vi "oa_TV Average methods(1Chan).vi"(5 "Window size":i16=10, 7 "Enum":T1(ring)=enum."Moving average", 9 "Revulotion index":i32, 10 "Angle intervals":dbl[](array[numeric]), 11 "Array":dbl[][](array[numeric])) -> (3 "Angle intervals":dbl[](array[numeric]))   [LabVIEW 2017, in "SoundVib_Torsional.lvlib"]
uses:
  <vilib>/addons/Sound and Vibration/Order Analysis/Torsional Vibration/SoundVib_Torsional.lvlib
  <vilib>/Analysis/baseanly.llb/Mean (DBL).vi
  <vilib>/Analysis/NI_AALBase.lvlib
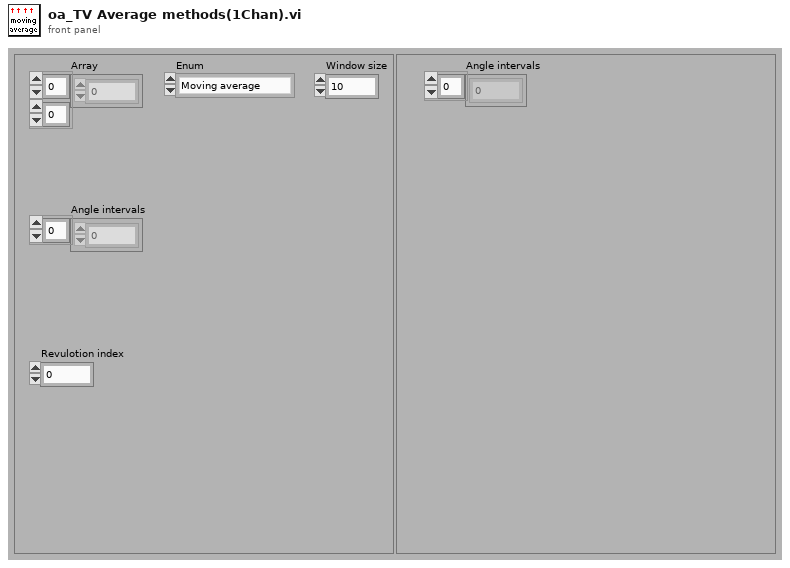
[diagram p1: front panel]
types:
  T1 = enum16{"Exponential average", "Moving average", "Current"}
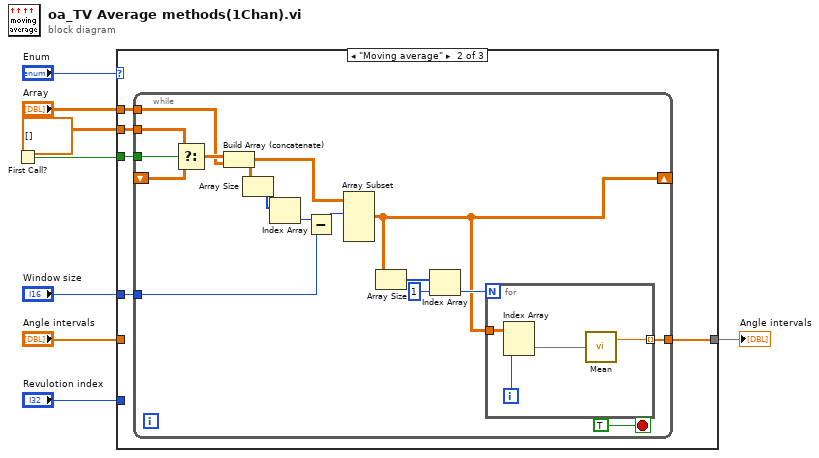
[diagram p0: block diagram]
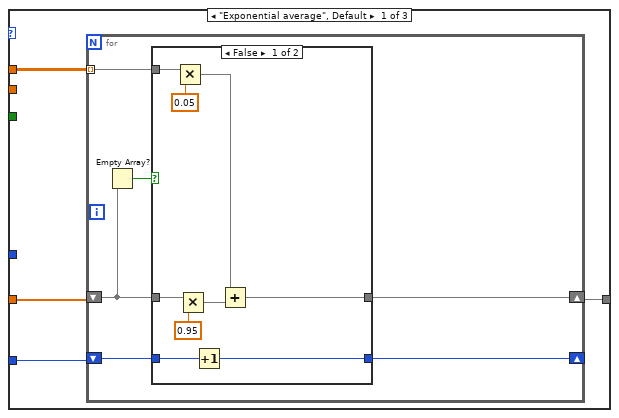
[diagram p2: hidden frame]
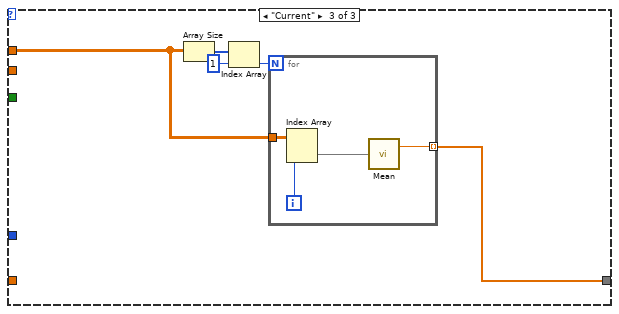
[diagram p4: hidden frame]
diagram:
  n1 = First Call?() -> (First Call?: T/F=w2:bool)
  n2 = case shown="\"Moving average\"" "Enum" {
    tunnel: "Array" -> [w12 w34 w56]
    tunnel: "Angle intervals" -> [w11 _ _]
    tunnel: [w10 w30 w55] -> w6
    tunnel: "Revulotion index" -> [w9 _ _]
    tunnel: "Window size" -> [_ w33 _]
    tunnel: w2 -> [_ w32 _]
    tunnel: dbl[][] [] ("Array") -> [_ w31 _]
    frame "Exponential average", Default {
      n3 = for {
        tunnel: w12 -> [w14] mode=indexing
        shift-right: [w17] -> _
        shift-left: w9 -> [w18]
        shift-right: [w13] -> w10
        shift-left: w11 -> [w16]
        n4 = Empty Array?(array=w16) -> (empty?=w15:bool)
        n5 = case shown="False" w15 {
          tunnel: [w19 w29] -> w13
          tunnel: w16 -> [w27 _]
          tunnel: w18 -> [w26 w28]
          tunnel: [w25 w28] -> w17
          tunnel: w14 -> [w22 w29]
          frame False {
            n6 = Multiply(x=w22, y=0.05 ("x+1")) -> (x*y=w20:dbl[])
            n7 = Multiply(x=w27, y=0.95 ("x+1")) -> (x*y=w24:dbl[])
            n8 = Increment(x=w26) -> (x+1=w25:i32)
            n9 = Add(x=w20, y=w24) -> (x+y=w19:dbl[])
          }
          frame True {
          }
        }
      }
    }
    frame "Moving average" {
      n10 = while {
        tunnel: w34 -> [w46]
        tunnel: w33 -> [w41]
        tunnel: w32 -> [w50]
        tunnel: w31 -> [w49]
        shift-right: [w36] -> _
        shift-left: _ -> [w48]
        tunnel: [w35] -> w30
        stop <- TRUE stop-if-true
        n11 = Select(t=w49, s=w50, f=w48) -> (s? t:f=w47:dbl[][])
        n12 = Build Array (concatenate)(w47, w46) -> (w44:dbl[][])
        n13 = Array Size(array=w44) -> (size(s)=w43:i32[])
        n14 = Index Array(array=w43) -> (element=w42:i32)  [unwired: 1 in]
        n15 = Subtract(x=w42, y=w41) -> (x-y=w40:i32)
        n16 = Array Subset(array=w44, index (row)=w40) -> (w36:dbl[][])  [unwired: 3 in]
        n17 = Array Size(array=w36) -> (size(s)=w39:i32[])
        n18 = Index Array(array=w39, index=1) -> (element=w37:i32)
        n19 = for {
          N: w37 -> [_]
          tunnel: w36 -> [w54]
          tunnel: [w51] -> w35 mode=indexing
          i -> [w53]
          n20 = Index Array(array=w54, index (col)=w53) -> (element=w52:dbl[])  [unwired: 1 in]
          n21 = call-poly <vilib>:"Mean.vi"("X"=w52) -> ("mean"=w51:dbl)  [unwired: 1 out]
        }
      }
    }
    frame "Current" {
      n22 = Array Size(array=w56) -> (size(s)=w59:i32[])
      n23 = Index Array(array=w59, index=1) -> (element=w57:i32)
      n24 = for {
        N: w57 -> [_]
        tunnel: w56 -> [w63]
        tunnel: [w60] -> w55 mode=indexing
        i -> [w62]
        n25 = Index Array(array=w63, index (col)=w62) -> (element=w61:dbl[])  [unwired: 1 in]
        n26 = call-poly <vilib>:"Mean.vi"("X"=w61) -> ("mean"=w60:dbl)  [unwired: 1 out]
      }
    }
  }
  "Angle intervals" <- w6
